vi "remove_package.vi"(8 "error in (no error)":errorcluster, 10 "package_manager":string="nipm", 11 "dragon_file_path":path=path "C:/Projects/labview-project-load-tools/rust_src/toml_edit_dll/lv_src/test.toml") -> ()   [LabVIEW 2020]
uses:
  dragon_toml_32.dll
panel:
  out "removed":bool
  in  "package_name":string="ni-daqmx"
  out "error out":errorcluster
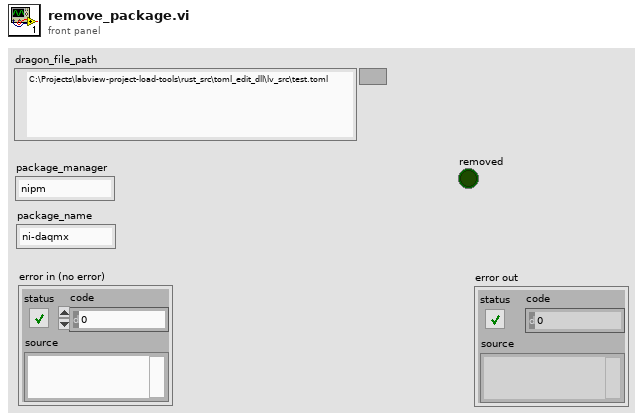
[diagram p1: front panel]
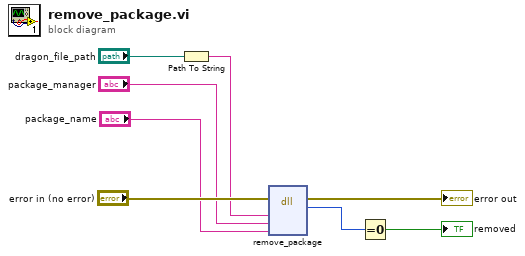
[diagram p0: block diagram]
diagram:
  n1 = Path To String(path="dragon_file_path") -> (string=w5:string)
  n2 = dll-call lib="C:/Projects/labview-project-load-tools/rust_src/toml_edit_dll/lv_src/dragon_toml_*.dll" fn="remove_package"(error in="error in (no error)", "file_path"=w5, "package_manager"="package_manager", "package_name"="package_name") -> (error out=→"error out":errorcluster, "result"=w2:i32)  [unwired: 5 in, 1 out]
  n3 = Equal To 0?(x=w2) -> (x = 0?=→"removed":bool)
